vi "Assymetric_Arbitrary_Function_Generator.vi"(7 "Desination Folder":path=path "C:/Users/Nick/Desktop", 8 "Limits":dbl[](array[numeric]), 9 "Frequency":dbl, 10 "Amplitude":dbl, 11 "Sample Length":i32) -> (1 "Arbitary Function":cluster{"xi used":dbl[], "yi":dbl[]}(graph), 2 "Amplitude":dbl, 3 "Offset":dbl)   [LabVIEW 2011]
uses:
  <vilib>/Analysis/baseanly.llb/Scale 1D.vi
  <vilib>/Analysis/1siggen.llb/Ramp Pattern by Samples.vi
  <vilib>/Analysis/NI_AALBase.lvlib
  <vilib>/Analysis/NI_AALPro.lvlib
  <vilib>/gmath/NI_Gmath.lvlib
panel:
  out "Residual":dbl
  out "Iterations":i32
  in  "Tolerance":dbl
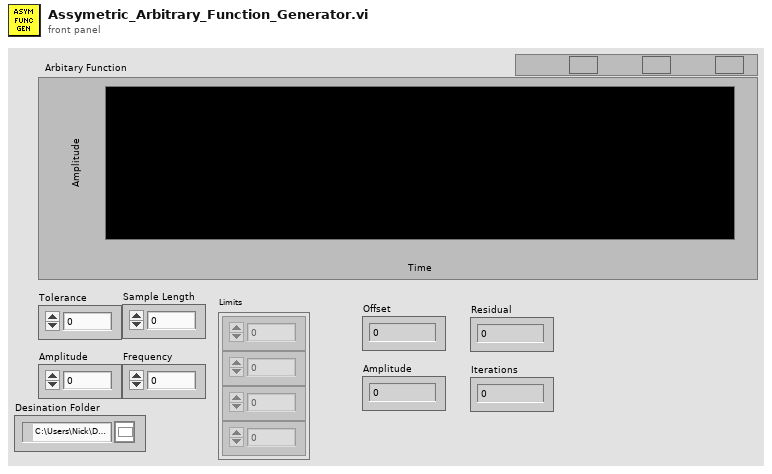
[diagram p1: front panel]
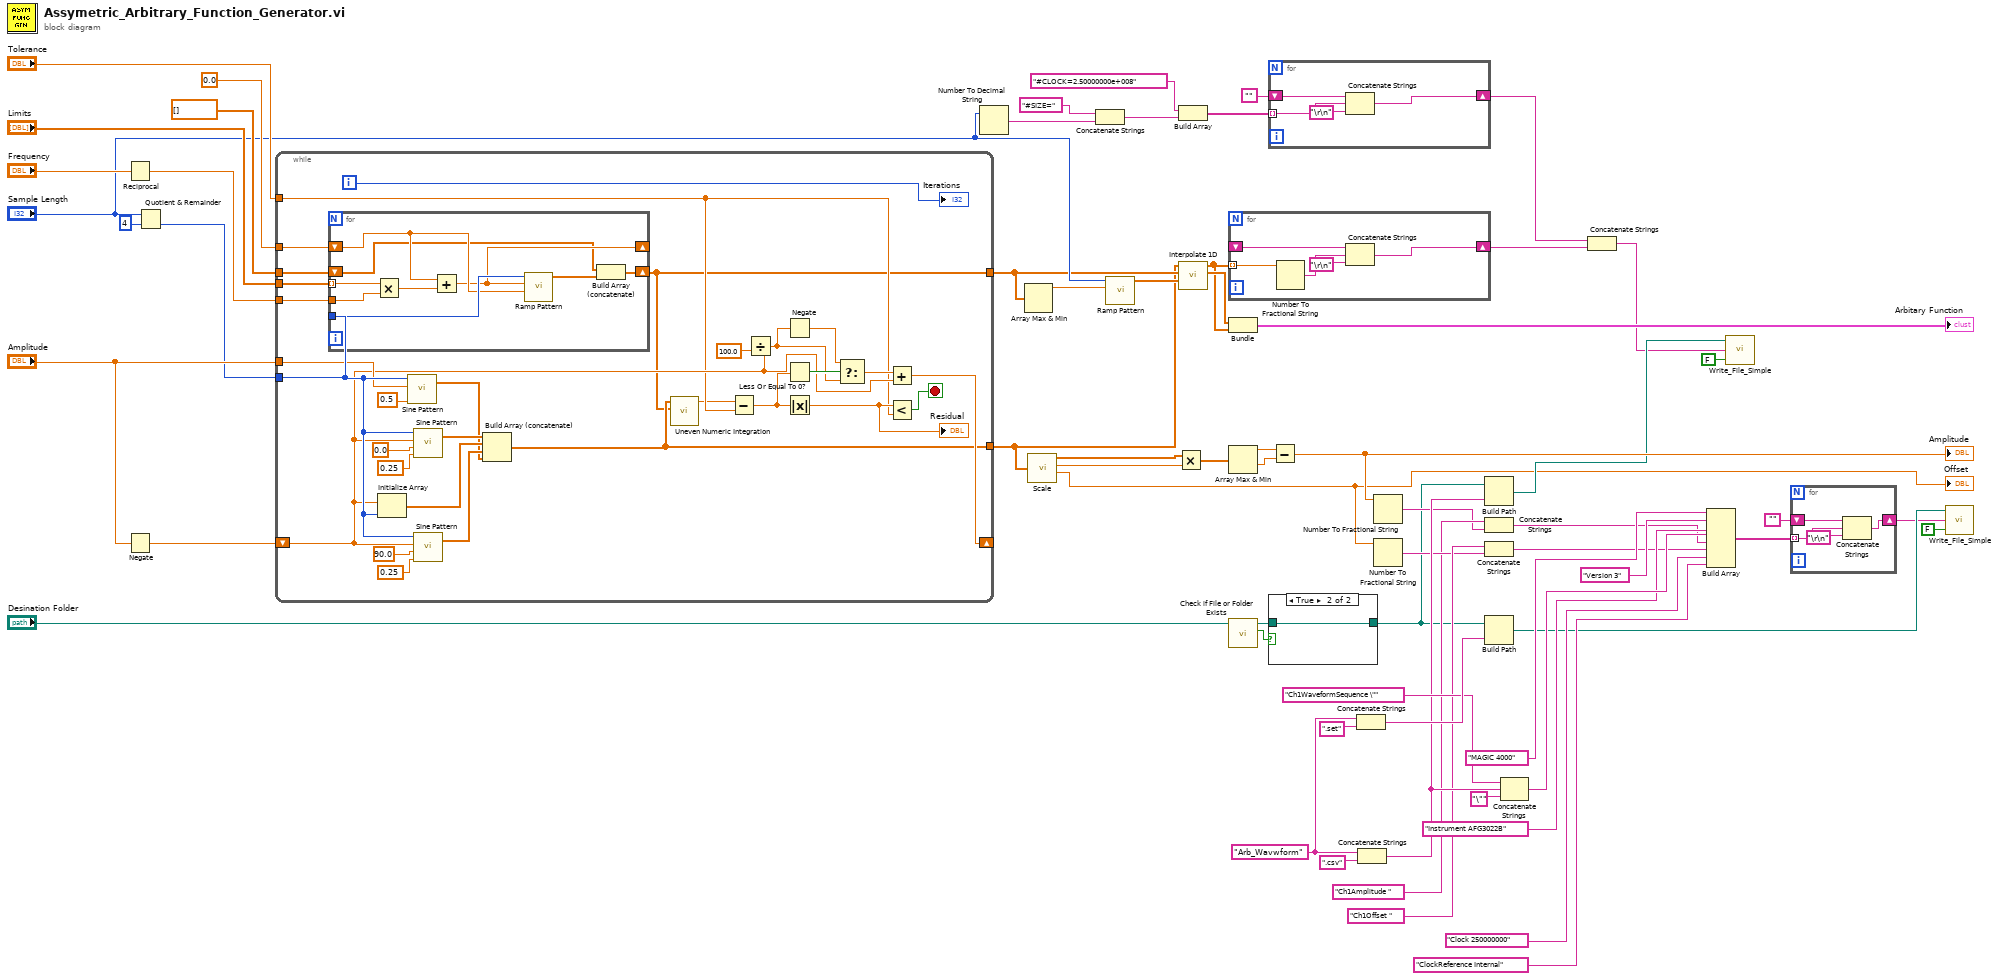
[diagram p0: block diagram]
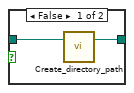
[diagram p2: hidden frame]
diagram:
  w51 = "Arb_Wavwform"
  n1 = Reciprocal(x="Frequency") -> (1/x=w57:dbl)
  n2 = Negate(x="Amplitude") -> (-x=w59:dbl)
  n3 = Quotient & Remainder(x="Sample Length", y=4) -> (floor(x/y)=w56:i32)  [unwired: 1 out]
  n4 = while {
    tunnel: 0.0 ("start") -> [w85]
    tunnel: dbl[] [] -> [w84]
    tunnel: [w65] -> w25
    tunnel: "Limits" -> [w83]
    tunnel: w56 -> [w82]
    tunnel: [w66] -> w12
    tunnel: "Amplitude" -> [w80]
    tunnel: "Tolerance" -> [w70]
    shift-right: [w73] -> _
    shift-left: w59 -> [w77]
    tunnel: w57 -> [w68]
    i -> [w81]
    stop <- w69 stop-if-true
    n5 = for {
      tunnel: w83 -> [w97] mode=indexing
      shift-right: [w101] -> _
      shift-left: w85 -> [w102]
      tunnel: w82 -> [w103]
      shift-right: [w98] -> w65
      shift-left: w84 -> [w100]
      tunnel: w68 -> [w96]
      n6 = Multiply(x=w97, y=w96) -> (x*y=w95:dbl)
      n7 = Add(x=w102, y=w95) -> (x+y=w101:dbl)
      n8 = call-poly <vilib>:"Ramp Pattern.vi"("start"=w102, "end"=w101, "samples"=w103) -> ("Ramp Pattern"=w99:dbl[])  [unwired: 7 in, 1 out]
      n9 = Build Array (concatenate)(w100, w99) -> (w98:dbl[])
    }
    n10 = Initialize Array(w77, w82) -> (w91:dbl[])
    n11 = call <vilib>:"Sine Pattern.vi"("cycles"=0.5, "amplitude"=w80, "samples"=w82) -> ("Sinusoidal Pattern"=w87:dbl[])  [unwired: 1 in, 1 out]
    n12 = call <vilib>:"Sine Pattern.vi"("cycles"=0.25, "phase(degrees)"=0.0 ("phase(degrees) 2"), "amplitude"=w77, "samples"=w82) -> ("Sinusoidal Pattern"=w93:dbl[])  [unwired: 1 out]
    n13 = call <vilib>:"Sine Pattern.vi"("cycles"=0.25, "phase(degrees)"=90.0, "amplitude"=w77, "samples"=w82) -> ("Sinusoidal Pattern"=w90:dbl[])  [unwired: 1 out]
    n14 = Build Array (concatenate)(w93, w91, w90, w87) -> (w66:dbl[])
    n15 = call <vilib>:"Uneven Numeric Integration.vi"("T"=w65, "X"=w66) -> ("result"=w67:dbl)  [unwired: 8 in, 1 out]
    n16 = Subtract(x=w67, y=w70) -> (x-y=w72:dbl)
    n17 = Divide(x=w77, y=100.0) -> (x/y=w75:dbl)
    n18 = Negate(x=w75) -> (-x=w74:dbl)
    n19 = Less Or Equal To 0?(x=w72) -> (x <= 0?=w79:bool)
    n20 = Absolute Value(x=w72) -> (abs(x)=w71:dbl)
    "Residual" <- w71
    n21 = Select(t=w74, s=w79, f=w75) -> (s? t:f=w78:dbl)
    n22 = Add(x=w78, y=w77) -> (x+y=w73:dbl)
    n23 = Less?(x=w71, y=w70) -> (x < y?=w69:bool)
    "Iterations" <- w81
  }
  n24 = Number To Decimal String(number="Sample Length") -> (decimal integer string=w45:string)  [unwired: 1 in]
  n25 = Array Max & Min(array=w25) -> (max value=w53:dbl)  [unwired: 3 out]
  n26 = call-poly <vilib>:"Scale.vi"("X"=w12) -> ("Y=(X-offset)/scale"=w24:dbl[], "scale"=w26:dbl, "offset"=w5:dbl)  [unwired: 1 out]
  "Offset" <- w5
  n27 = Concatenate Strings("#SIZE=" ("string"), w45) -> (w44:string)
  n28 = call-poly <vilib>:"Ramp Pattern.vi"("end"=w53, "samples"="Sample Length") -> ("Ramp Pattern"=w54:dbl[])  [unwired: 8 in, 1 out]
  n29 = Multiply(x=w24, y=w26) -> (x*y=w23:dbl[])
  n30 = Build Array("#CLOCK=2.50000000e+008" ("string"), w44) -> (w43:string[])
  n31 = call <vilib>:"Interpolate 1D.vi"("xi"=w54, "X"=w25, "Y"=w12) -> ("xi used"=w16:dbl[], "yi"=w14:dbl[])  [unwired: 6 in, 1 out]
  n32 = for {
    shift-right: [w107] -> w13
    shift-left: _ -> [w106]
    tunnel: w14 -> [w105] mode=indexing
    n33 = Number To Fractional String(number=w105) -> (F-format string=w104:string)  [unwired: 3 in]
    n34 = Concatenate Strings(w106, w104, "\r\n") -> (w107:string)
  }
  n35 = Bundle("xi used"=w16, "yi"=w14) -> (→"Arbitary Function":cluster{"xi used":dbl[], "yi":dbl[]})  [unwired: 1 in]
  n36 = Array Max & Min(array=w23) -> (max value=w22:dbl, min value=w21:dbl)  [unwired: 2 out]
  n37 = call <vilib>:"Check if File or Folder Exists.vi"("path"="Desination Folder") -> ("file or folder exists?"=w2:bool, "dup path"=w3:path)  [unwired: 8 in, 1 out]
  n38 = for {
    tunnel: w43 -> [w112] mode=indexing
    shift-right: [w110] -> w42
    shift-left: "" -> [w109]
    n39 = Concatenate Strings(w109, w112, "\r\n") -> (w110:string)
  }
  n40 = case shown="True" w2 {
    tunnel: w3 -> [w114 w115]
    tunnel: [w113 w115] -> w1
    frame False {
      n41 = call "Create_directory_path.vi"("Path name"=w114) -> ("Path name Out"=w113:path)  [unwired: 1 in, 1 out]
    }
    frame True {
    }
  }
  n42 = Subtract(x=w22, y=w21) -> (x-y=w20:dbl)
  "Amplitude" <- w20
  n43 = Concatenate Strings(w51, ".set" ("string")) -> (w49:string)
  n44 = Concatenate Strings(w51, ".csv" ("string")) -> (w40:string)
  n45 = Number To Fractional String(number=w20) -> (F-format string=w18:string)  [unwired: 3 in]
  n46 = Number To Fractional String(number=w5) -> (F-format string=w28:string)  [unwired: 3 in]
  n47 = Build Path(base path=w1, name or relative path=w40) -> (appended path=w8:path)
  n48 = Concatenate Strings("Ch1Amplitude " ("string"), w18) -> (w17:string)
  n49 = Concatenate Strings("Ch1Offset " ("string"), w28) -> (w27:string)
  n50 = Build Path(base path=w1, name or relative path=w49) -> (appended path=w11:path)
  n51 = Concatenate Strings("Ch1WaveformSequence \"" ("string"), w40, "\"" ("string")) -> (w38:string)
  n52 = Concatenate Strings(w42, w13) -> (w7:string)
  n53 = Build Array("MAGIC 4000" ("string"), "Version 3" ("string"), "Instrument AFG3022B" ("string"), w38, w17, w27, "Clock 250000000" ("string"), "ClockReference Internal" ("string")) -> (w32:string[])
  n54 = call "Write_File_Simple.vi"("append to file? (new file:F)"=FALSE, "character string"=w7, "file path"=w8) -> ()  [unwired: 2 out]
  n55 = for {
    tunnel: w32 -> [w119] mode=indexing
    shift-right: [w117] -> w10
    shift-left: "" -> [w116]
    n56 = Concatenate Strings(w116, w119, "\r\n") -> (w117:string)
  }
  n57 = call "Write_File_Simple.vi"("append to file? (new file:F)"=FALSE, "character string"=w10, "file path"=w11) -> ()  [unwired: 2 out]
